vi "Error Calculations.vi"(8 "Accepted":dbl, 11 "Measured":dbl) -> (3 "Error":dbl)   [LabVIEW 2014]
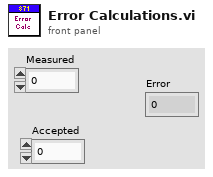
[diagram p1: front panel]
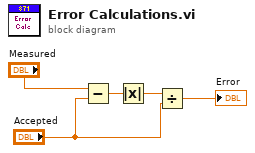
[diagram p0: block diagram]
diagram:
  n1 = Subtract(x="Measured", y="Accepted") -> (x-y=w4:dbl)
  n2 = Absolute Value(x=w4) -> (abs(x)=w3:dbl)
  n3 = Divide(x=w3, y="Accepted") -> (x/y=→"Error":dbl)
